vi "rotate old test.vi"   [LabVIEW 2019]
uses:
  <vilib>/Platform/TimedLoop/XDataNode/timing_clust.ctl
  <vilib>/Platform/TimedLoop/XDataNode/nitl_modes.ctl
  <vilib>/Platform/TimedLoop/XDataNode/wakeup.ctl
  <vilib>/platform/TimedLoop/XDataNode/XDataNode.xnode
  <vilib>/Platform/TimedLoop/XDataNode/XDNodeRunTimeDep.lvlib
types:
  T1 = typedef "XDNodeRunTimeDep.lvlib/timing_clust.ctl" = cluster{"Expected End [f-1]":u64, "Actual End [f-1]":u64, "Finished Late? [f-1]":bool, "Expected End [i-1]":u64, "Actual End [i-1]":u64, "Finished Late? [i-1]":bool, "Expected Start [i]":u64, "Actual Start [i]":u64, "Expected Start [f]":u64, "Actual Start [f]":u64, "Source Name":string, "Structure Name":string, "Period":i64, "Deadline":i64, "Offset":i64, "Start":i64, "Priority":i32, "Timeout":i32, "Mode":T2, "Wakeup Reason":T3, "Error":errorcluster, "Source Type":string, "Secondary Source Type":string, "Global End Time":u64, "Global Start Time":u64, "Frame Duration":u64, "Iteration Duration":u64, "Assigned CPU":i32, "I/O Scan Engine Mode":u32}
  T2 = typedef "XDNodeRunTimeDep.lvlib/nitl_modes.ctl" = enum32{"No Change", "Process missed periods, maintain original phase", "Discard missed periods, maintain original phase", "Process missed periods, ignore original phase", "Discard missed periods, ignore original phase"}
  T3 = typedef "XDNodeRunTimeDep.lvlib/wakeup.ctl" = enum32{"Normal", "Aborted", "Asynchronous wakeup", "Timing source error", "Timed loop error", "Timeout"}
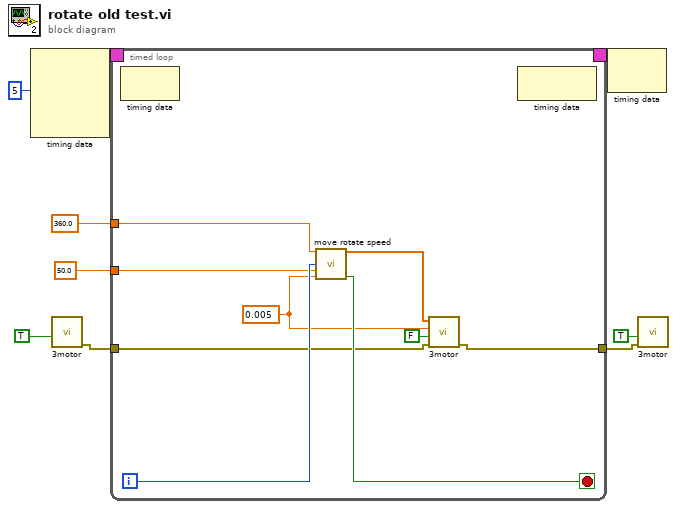
[diagram p0: block diagram]
diagram:
  n1 = node-c288(i64 5 ("Period")) -> (w9:T1)  [unwired: 3 in]
  n2 = call "3motor.vi"("Reset"=TRUE) -> ("error out"=w4:errorcluster)  [unwired: 10 in]
  n3 = timed-loop {
    timing: w9 -> [_]
    timing-out: [_] -> w8
    tunnel: 50.0 -> [w16]
    tunnel: 360.0 ("rotate degree") -> [w15]
    tunnel: w4 -> [w11]
    tunnel: [w10] -> w1
    i -> [w18]
    stop <- w17 stop-if-true
    w13 = 0.005 ("dt(s)")
    n4 = node-c288() -> ()  [unwired: 1 in, 1 out]
    n5 = call "move rotate speed.vi"("rotate degree"=w15, "i"=w18, "speed"=w16, "dt(s)"=w13) -> ("speed out"=w14:dbl[], "complet?"=w17:bool)  [unwired: 6 in, 4 out]
    n6 = call "3motor.vi"("error in (no error)"=w11, "Reset"=FALSE, "dt(s)"=w13, "Motor speed"=w14) -> ("error out"=w10:errorcluster)  [unwired: 7 in]
    n7 = node-c288() -> ()  [unwired: 1 in, 1 out]
  }
  n8 = node-c288(w8) -> ()  [unwired: 1 out]
  n9 = call "3motor.vi"("error in (no error)"=w1, "Reset"=TRUE) -> ()  [unwired: 9 in, 1 out]
